vi "Set File Position.vi"(7 "New Position (1)":i32=1, 8 "error in (no error)":errorcluster, 9 "Start Position (1: Current Position)":i32(ring)=1 items=["Beginning of File", "Current Position", "End of file"], 10 "File Variable":string, 11 "VISA resource name":refnum<visa-resource-name>) -> (0 "error out":errorcluster, 1 "Error Message":string, 2 "Data Position":dbl, 3 "VISA resource name out":refnum<visa-resource-name>)   [LabVIEW 2015, in "Keithley 2600 Series.lvlib"]
doc: "Sets file's current position."
uses:
  Keithley 2600 Series.lvlib
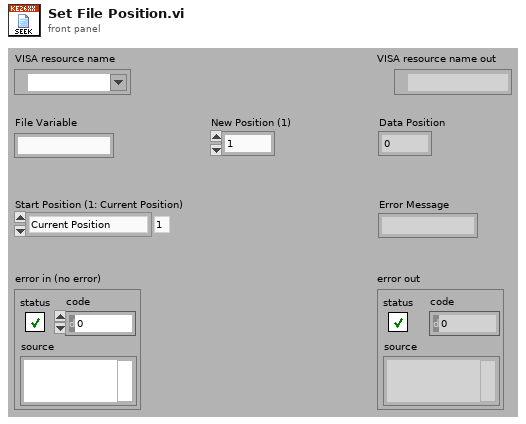
[diagram p1: front panel]
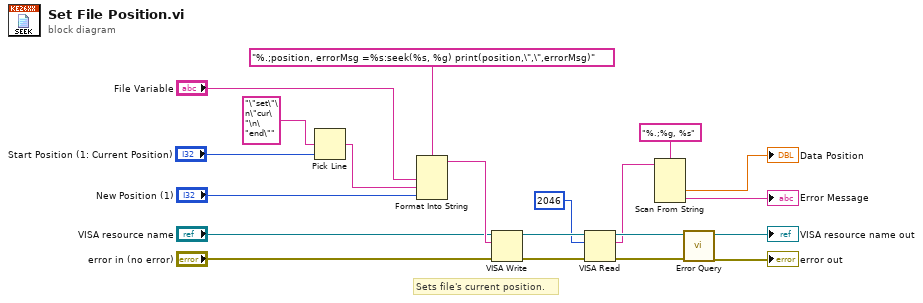
[diagram p0: block diagram]
diagram:
  # "Sets file's current position."
  n1 = Pick Line(multi-line string="\"set\"\n\"cur\"\n\"end\"", line index="Start Position (1: Current Position)") -> (output string=w10:string)  [unwired: 1 in]
  n2 = Format Into String(format string="%.;position, errorMsg =%s:seek(%s, %g) print(position,\",\",errorMsg)", "File Variable", w10, "New Position (1)") -> (resulting string=w17:string)  [unwired: 2 in, 1 out]
  n3 = VISA Write(VISA resource name="VISA resource name", write buffer=w17, error in (no error)="error in (no error)") -> (VISA resource name out=w9:refnum<visa-resource-name>, error out=w8:errorcluster)  [unwired: 1 out]
  n4 = VISA Read(VISA resource name=w9, byte count=u32 2046, error in (no error)=w8) -> (VISA resource name out=w7:refnum<visa-resource-name>, read buffer=w5:string, error out=w6:errorcluster)  [unwired: 1 out]
  n5 = Scan From String(format string="%.;%g, %s", input string=w5) -> (output 1=→"Data Position":dbl, output 2=→"Error Message":string)  [unwired: 4 in, 3 out]
  n6 = call "Error Query.vi"("error in (no error)"=w6, "VISA resource name"=w7) -> ("error out"=→"error out":errorcluster, "VISA resource name out"=→"VISA resource name out":refnum<visa-resource-name>)  [unwired: 6 in, 2 out]
